vi "Obtain Notifier Registry.vi"(8 "error in (no error)":errorcluster) -> (0 "error out":errorcluster, 3 "Notifier Registry":refnum<notifier>)   [LabVIEW 2021]
doc: "This VI initialized the queue registry. It utilizes the first call function to obtain a new queue registry, then every call thereafter uses the same registry reference."
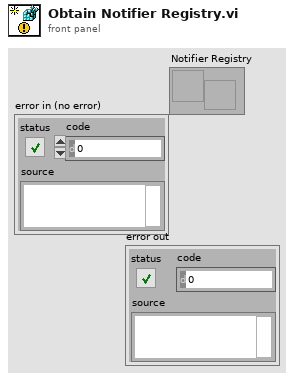
[diagram p1: front panel]
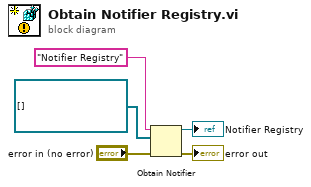
[diagram p0: block diagram]
diagram:
  n1 = Obtain Notifier(name (unnamed)="Notifier Registry", notification data type=refnum<notifier>[] [], error in (no error)="error in (no error)") -> (notifier out=→"Notifier Registry":refnum<notifier>, error out=→"error out":errorcluster)  [unwired: 1 in, 1 out]
